vi "Close People Tracking Refs.vi"(8 "error in (no error)":errorcluster, 11 "ball tracking refs":T1={"acquired image"=refnum, "threshold image"=refnum, "Video Handle out"=0, "Kinect Handle"=0, "Video and Depth config"={"Video Resolution"=enum."FREENECT_RESOLUTION_LOW", "Video Format"=enum."FREENECT_VIDEO_RGB", "Depth Format"=enum."FREENECT_DEPTH_11BIT", "Depth Resolution"=enum."FREENECT_RESOLUTION_MEDIUM"}}) -> (0 "error out":errorcluster)   [LabVIEW 2014]
doc: "Close the camera session, and dispose the image buffers."
uses:
  Ball Tracking Image Refs.ctl
  <vilib>/vision/Image Controls.llb/IMAQ Image.ctl
  KinectProject/subVIs/Video Resolution Control.ctl
  KinectProject/subVIs/Video Format Control.ctl
  KinectProject/subVIs/Depth Format Control.ctl
  KinectProject/subVIs/Depth Resolution Control.ctl
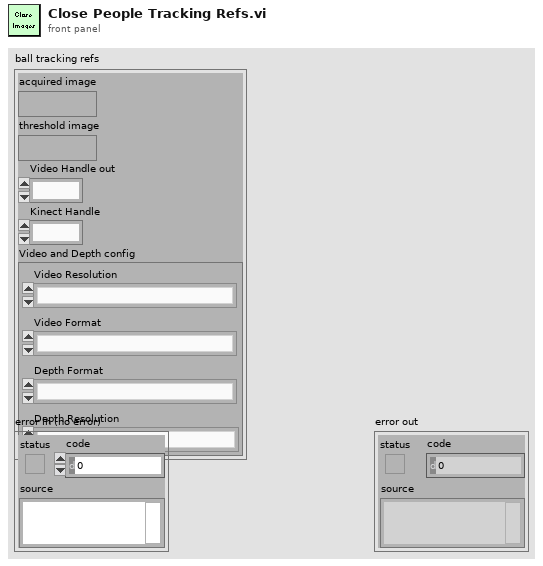
[diagram p1: front panel]
types:
  T1 = typedef "Ball Tracking Image Refs.ctl" = cluster{"acquired image":T2, "threshold image":T2, "Video Handle out":i64, "Kinect Handle":i64, "Video and Depth config":cluster{"Video Resolution":T3, "Video Format":T4, "Depth Format":T5, "Depth Resolution":T6}}
  T2 = typedef "IMAQ Image.ctl" = refnum<image>
  T3 = typedef "Video Resolution Control.ctl" = enum32{"FREENECT_RESOLUTION_LOW", "FREENECT_RESOLUTION_MEDIUM", "FREENECT_RESOLUTION_HIGH"}
  T4 = typedef "Video Format Control.ctl" = enum32{"FREENECT_VIDEO_RGB", "FREENECT_VIDEO_BAYER", "FREENECT_VIDEO_IR_8BIT", "FREENECT_VIDEO_IR_10BIT", "FREENECT_VIDEO_IR_10BIT_PACKED", "FREENECT_VIDEO_YUV_RGB", "FREENECT_VIDEO_YUV_RAW"}
  T5 = typedef "Depth Format Control.ctl" = enum32{"FREENECT_DEPTH_11BIT", "FREENECT_DEPTH_10BIT", "FREENECT_DEPTH_11BIT_PACKED", "FREENECT_DEPTH_10BIT_PACKED", "FREENECT_DEPTH_REGISTERED", "FREENECT_DEPTH_MM"}
  T6 = typedef "Depth Resolution Control.ctl" = enum16{"FREENECT_RESOLUTION_TINY", "FREENECT_RESOLUTION_LOW", "FREENECT_RESOLUTION_MEDIUM"}
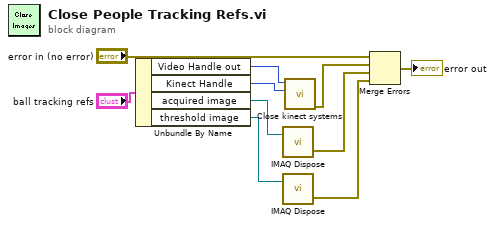
[diagram p0: block diagram]
diagram:
  n1 = Unbundle By Name("ball tracking refs") -> ("Video Handle out"=w3:i64, "Kinect Handle"=w2:i64, "acquired image"=w9:T2, "threshold image"=w8:T2)
  n2 = call "IMAQ Dispose"("Image"=w9) -> ("error out"=w7:errorcluster)  [unwired: 5 in]
  n3 = call "IMAQ Dispose"("Image"=w8) -> ("error out"=w6:errorcluster)  [unwired: 5 in]
  n4 = call "Close kinect systems.vi"("Kinect Handle"=w2, "Video handle in"=w3) -> ("error out"=w1:errorcluster)  [unwired: 9 in]
  n5 = Merge Errors("error in (no error)", w1, w7, w6) -> (→"error out":errorcluster)
